vi "SIMULACIJA.vi"() -> ()   [LabVIEW 2013]
panel:
  in  "Unesite trajanje pulsa u us":dbl
  out "NAPON":dynamicdata(graph)
  out "Izlazni napon u V":dbl
  out "Izmjerena udaljenost u cm":dbl
  in  "Stop":bool
  in  "Start":bool
  in  "Trajanje akvizicije u sec.":dbl
  out "DUŽINA":dynamicdata(graph)
  out "TRAJANJE IMPULSA":dynamicdata(graph)
  out "Vrijeme pulsa u us":dbl
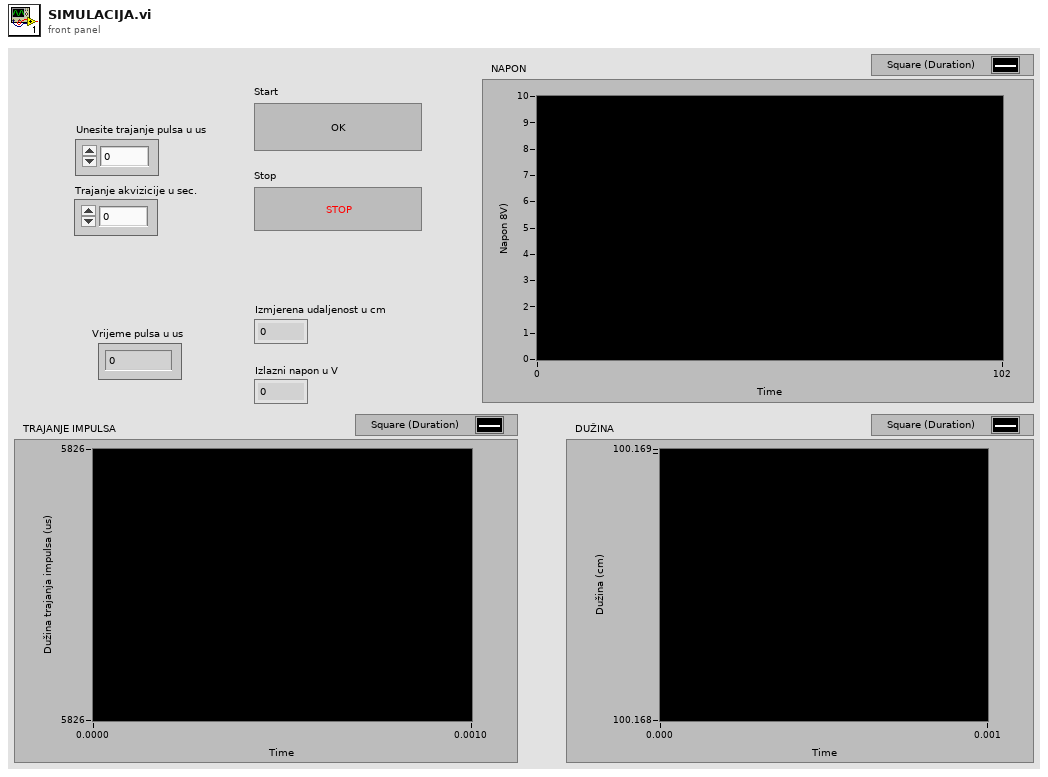
[diagram p1: front panel]
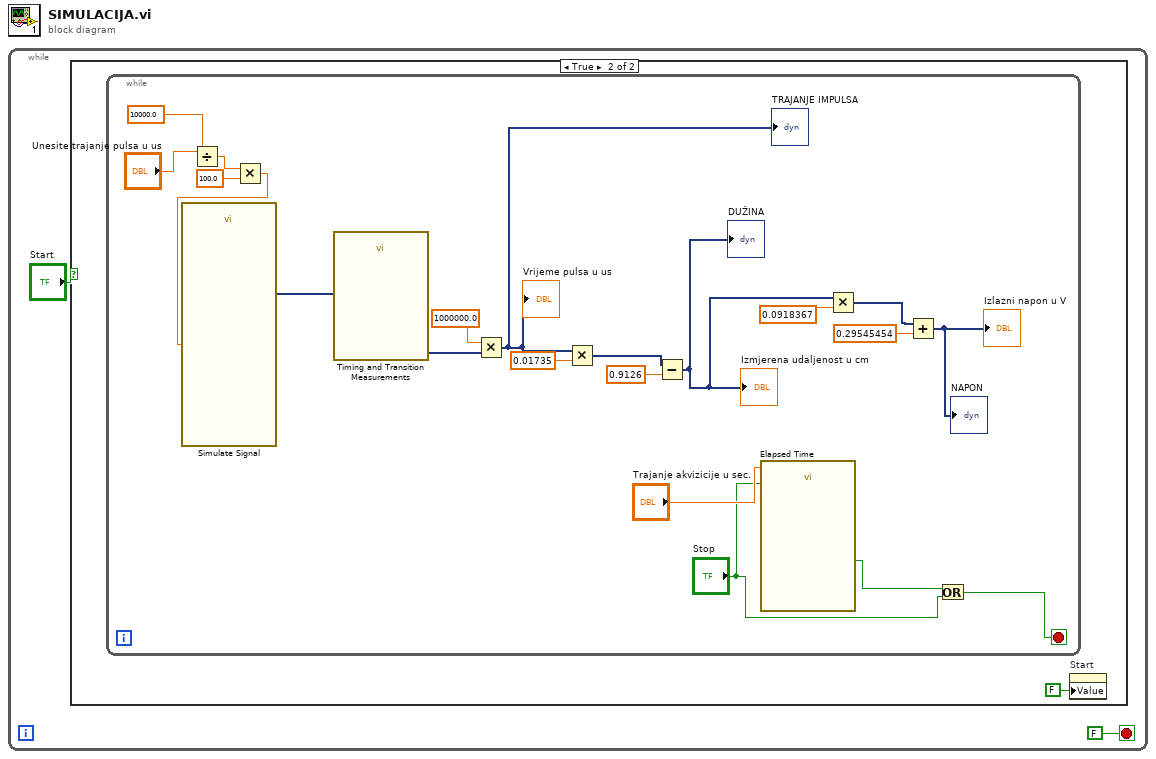
[diagram p0: block diagram]
diagram:
  n1 = while {
    stop <- FALSE stop-if-true
    n2 = case shown="True" "Start" {
      frame False {
      }
      frame True {
        n3 = while {
          stop <- w19 stop-if-true
          n4 = Divide(x="Unesite trajanje pulsa u us", y=10000.0) -> (x/y=w6:dbl)
          n5 = Multiply(x=w6, y=100.0) -> (x*y=w4:dbl)
          n6 = call "Simulate Signal"("Duty Cycle (%)"=w4) -> ("Square"=w9:dynamicdata)  [unwired: 13 in, 1 out]
          n7 = call "Timing and Transition Measurements"("Signals"=w9) -> ("Duration"=w24:dynamicdata)  [unwired: 9 in, 1 out]
          n8 = Multiply(x=1000000.0, y=w24) -> (x*y=w15:dynamicdata)
          "Vrijeme pulsa u us" <- w15
          "TRAJANJE IMPULSA" <- w15
          n9 = Multiply(x=w15, y=0.01735) -> (x*y=w17:dynamicdata)
          n10 = Subtract(x=w17, y=0.9126) -> (x-y=w14:dynamicdata)
          "DUŽINA" <- w14
          "Izmjerena udaljenost u cm" <- w14
          n11 = call "Elapsed Time"("Time Target (s)"="Trajanje akvizicije u sec.", "Reset"="Stop") -> ("Time has Elapsed"=w21:bool)  [unwired: 10 in, 7 out]
          n12 = Multiply(x=w14, y=0.0918367) -> (x*y=w12:dynamicdata)
          n13 = Add(x=w12, y=0.29545454) -> (x+y=→"Izlazni napon u V" →"NAPON":dynamicdata)
          n14 = Or(x=w21, y="Stop") -> (x .or. y?=w19:bool)
        }
        n15 = property on="Start" class="Bool (strict)"("Value"=FALSE ("Start")) -> ()  [unwired: 2 in, 2 out]
      }
    }
  }
